vi "Get Satellite Data.vi"(8 "error in (no error)":errorcluster, 10 "Complete NMEA Sentences":string[](array[string]), 11 "VISA resource name":refnum<visa-resource-name>) -> (0 "error out":errorcluster, 1 "Satellite Data":cluster{i8, cluster{i32, i32, i32, i32}[]}[](array[cluster]), 2 "Complete NMEA Sentences (Copy)":string[](array[string]), 3 "VISA resource name out":refnum<visa-resource-name>)   [LabVIEW 2009]
doc: "Parses out the satellite data from all of the sentences that Read Raw.vi outputs, and passes through a complete copy of those sentences. Can be used in conjunction with other advanced \"Get\" VIs. See u-blox 5 Series Acquire and Chart GPS Advanced.vi for an example of how to use this VI.\n\nNote that the VISA Resource is not required, since this VI is a helper that does not actually interact with the device. The VISA Resource can be used, however, to clarify programming and maintain uniformity."
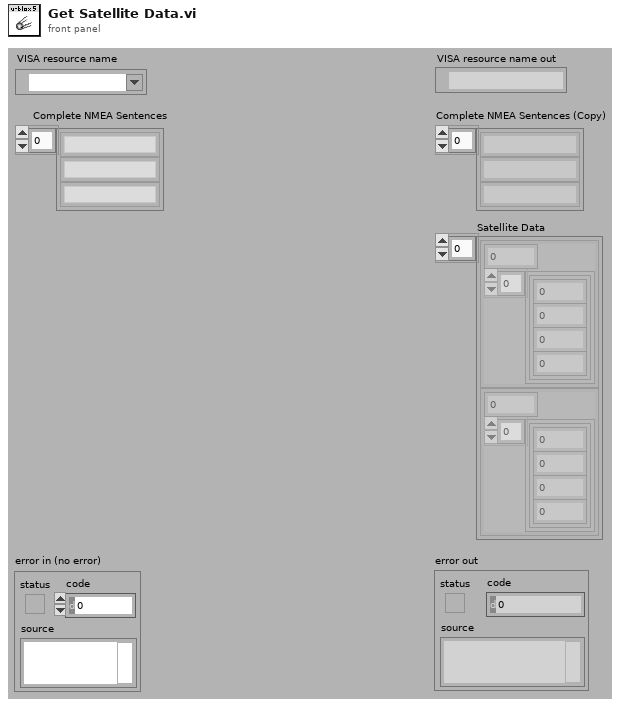
[diagram p1: front panel]
types:
  T1 = cluster{"# of Satellites":i8, "Satellite Data":cluster{i32, i32, i32, i32}[]}
  T2 = typedef "GSV Data.ctl" = cluster{"number of sentences for full data":cluster{"included?":bool, "number of sentences":i8}, "sentence number":cluster{"included?":bool, "number":i8}, "number of satellites in view":cluster{"included?":bool, "number of satellites":i8}, "satellite data":cluster{"included?":bool[], "data":cluster{"PRN number":i32, "elevation (deg)":i32, "azimuth (deg)":i32, "signal to noise ratio":i32}[]}}
  T3 = cluster{"PRN number":i32, "elevation (deg)":i32, "azimuth (deg)":i32, "signal to noise ratio":i32}[]
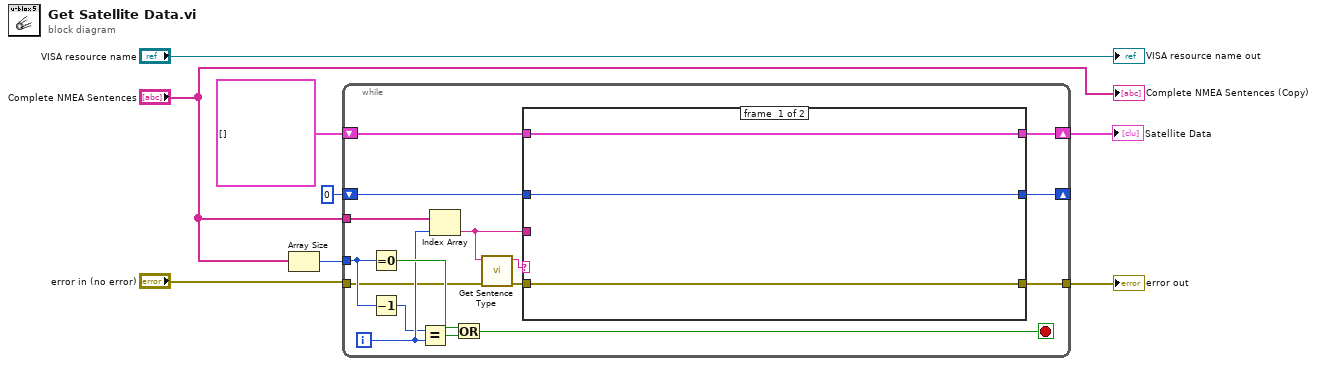
[diagram p0: block diagram]
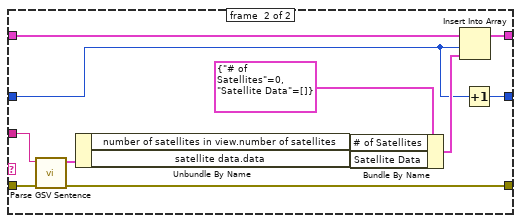
[diagram p2: hidden frame]
diagram:
  n1 = Array Size(array="Complete NMEA Sentences") -> (size(s)=w7:i32)
  n2 = while {
    tunnel: "Complete NMEA Sentences" -> [w24]
    shift-right: [w22] -> w1
    shift-left: cluster{i8, cluster{i32, i32, i32, i32}[]}[] [] -> [w21]
    tunnel: w7 -> [w18]
    tunnel: "error in (no error)" -> [w12]
    tunnel: [w23] -> w5
    shift-right: [w19] -> _
    shift-left: 0 -> [w20]
    i -> [w14]
    stop <- w16 stop-if-true
    n3 = Equal To 0?(x=w18) -> (x = 0?=w17:bool)
    n4 = Decrement(x=w18) -> (x-1=w13:i32)
    n5 = Equal?(x=w13, y=w14) -> (x = y?=w15:bool)
    n6 = Index Array(array=w24, index=w14) -> (element=w9:string)
    n7 = Or(x=w17, y=w15) -> (x .or. y?=w16:bool)
    n8 = call "Get Sentence Type.vi"("error in (no error)"=w12, "sentence"=w9) -> ("error out"=w11:errorcluster, "sentence type"=w10:string)  [unwired: 7 in, 1 out]
    n9 = case shown="\"\", Default" w10 {
      tunnel: w9 -> [_ w29]
      tunnel: w11 -> [w27 w30]
      tunnel: [w27 w31] -> w23
      tunnel: [w26 w39] -> w22
      tunnel: w21 -> [w26 w38]
      tunnel: w20 -> [w25 w32]
      tunnel: [w25 w37] -> w19
      frame #0 {
      }
      frame #1 {
        n10 = call "Parse GSV Sentence.vi"("error in (no error)"=w30, "GSV sentence"=w29) -> ("error out"=w31:errorcluster, "GSV data"=w28:T2)  [unwired: 8 in]
        n11 = Unbundle By Name(w28) -> ("number of satellites in view.number of satellites"=w33:i8, "satellite data.data"=w34:T3)
        n12 = Bundle By Name(cluster=T1 {"# of Satellites"=0, "Satellite Data"=[]}, "# of Satellites"=w33, "Satellite Data"=w34) -> (w36:T1)
        n13 = Insert Into Array(array=w38, index=w32, new element=w36) -> (w39:cluster{i8, cluster{i32, i32, i32, i32}[]}[])
        n14 = Increment(x=w32) -> (x+1=w37:i32)
      }
    }
  }
  "error out" <- w5
  "Satellite Data" <- w1
  "VISA resource name out" <- "VISA resource name"
  "Complete NMEA Sentences (Copy)" <- "Complete NMEA Sentences"
